vi "Drive.vi"() -> ()   [LabVIEW 2012]
uses:
  Robot Global Data.vi
  <vilib>/Rock Robotics/WPI/Joystick/WPI_JoystickGetSetRefNum.vi
  <vilib>/Rock Robotics/WPI/RobotDrive/WPI_RobotDriveGetSetRefNum.vi
  <vilib>/addons/control/pid/pid.llb/PID (DBL).vi
  <vilib>/addons/control/pid/NI_PID_pid.lvlib
panel:
  in  "PID gains":T1={"proportional gain (Kc)"=1.0, "integral time (Ti, min)"=0.01, "derivative time (Td, min)"=0.0} {"derivative time (Td, min)" format="%.3f"; "integral time (Ti, min)" format="%.3f"; "proportional gain (Kc)" format="%.3f"}
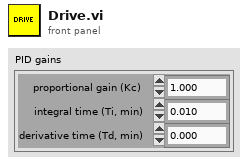
[diagram p1: front panel]
types:
  T1 = cluster{"proportional gain (Kc)":dbl, "integral time (Ti, min)":dbl, "derivative time (Td, min)":dbl}
  T2 = cluster{"Center Position":cluster{"X":dbl, "Y":dbl}, "Distance (ft)":dbl, "Center":bool}[]
  T3 = cluster{"Target Info[0]":cluster{"Center Position":cluster{"X":dbl, "Y":dbl}, "Distance (ft)":dbl, "Center":bool}, "Target Info[1]":cluster{"Center Position":cluster{"X":dbl, "Y":dbl}, "Distance (ft)":dbl, "Center":bool}, "Target Info[2]":cluster{"Center Position":cluster{"X":dbl, "Y":dbl}, "Distance (ft)":dbl, "Center":bool}, "Target Info[3]":cluster{"Center Position":cluster{"X":dbl, "Y":dbl}, "Distance (ft)":dbl, "Center":bool}, "Target Info[4]":cluster{"Center Position":cluster{"X":dbl, "Y":dbl}, "Distance (ft)":dbl, "Center":bool}, "Target Info[5]":cluster{"Center Position":cluster{"X":dbl, "Y":dbl}, "Distance (ft)":dbl, "Center":bool}, "Target Info[6]":cluster{"Center Position":cluster{"X":dbl, "Y":dbl}, "Distance (ft)":dbl, "Center":bool}, "Target Info[7]":cluster{"Center Position":cluster{"X":dbl, "Y":dbl}, "Distance (ft)":dbl, "Center":bool}, "Target Info[8]":cluster{"Center Position":cluster{"X":dbl, "Y":dbl}, "Distance (ft)":dbl, "Center":bool}}
  T4 = cluster{"Center Position":cluster{"X":dbl, "Y":dbl}, "Distance (ft)":dbl, "Center":bool}
  T5 = typedef "WPI_JoystickDevRef.ctl" = cluster{"Device":T6}
  T6 = typedef "WPI_JoystickDeviceEnum.ctl" = enum16{"USB 1", "USB 2", "USB 3", "USB 4", "Kinect 1", "Kinect 2"}
  T7 = typedef "WPI_JoystickButtonState.ctl" = cluster{"Button 1":bool, "Button 2":bool, "Button 3":bool, "Button 4":bool, "Button 5":bool, "Button 6":bool, "Button 7":bool, "Button 8":bool, "Button 9":bool, "Button 10":bool, "Button 11":bool, "Button 12":bool}
  T8 = cluster{"axis 1 (x)":dbl, "axis 2 (y)":dbl, "axis 3 (throttle)":dbl, "axis 4":dbl, "axis 5":dbl, "axis 6":dbl}
  T9 = typedef "WPI_RobotDriveDevRef.ctl" = cluster{"DevStatus":errorcluster, "Motors[]":T10[], "Square Inputs":bool, "Max Output":dbl, "Isochronous":bool}
  T10 = typedef "WPI_MotorControlDeviceRef.ctl" = cluster{"DeviceStatus":errorcluster, "Type":enum16{"PWM", "CAN"}, "PWM":cluster{"Digital Module":T11, "PWM Channel":T12, "DeadBand":T13}, "CAN":cluster{"Device Number":u8, "Control Mode":T14, "Semaphore":T15, "Max Vout":dbl}, "Invert":bool, "TransformRef":T16, "InvTransformRef":T16}
  T11 = typedef "FPGA_TypedefDigitalModule.ctl" = enum16{"Digital Module 1", "Digital Module 2"}
  T12 = typedef "FPGA_DIOPWMChannel.ctl" = enum8{"PWM 1", "PWM 2", "PWM 3", "PWM 4", "PWM 5", "PWM 6", "PWM 7", "PWM 8", "PWM 9", "PWM 10", "Invalid"}
  T13 = typedef "WPI_PWMDeadband.ctl" = cluster{"Name":string, "maxPositivePwm":i32, "minPositivePwm":i32, "centerPwm":i32, "maxNegativePwm":i32, "minNegativePwm":i32, "angularRange":u16}
  T14 = typedef "WPI_CANJaguar_ControlMode.ctl" = enum8{"Percent VBus", "Current", "Speed", "Position", "Voltage"}
  T15 = typedef "Semaphore RefNum" = refnum<k1>
  T16 = typedef "WPI_PWMTransform_ConPane.ctl" = refnum<vi>
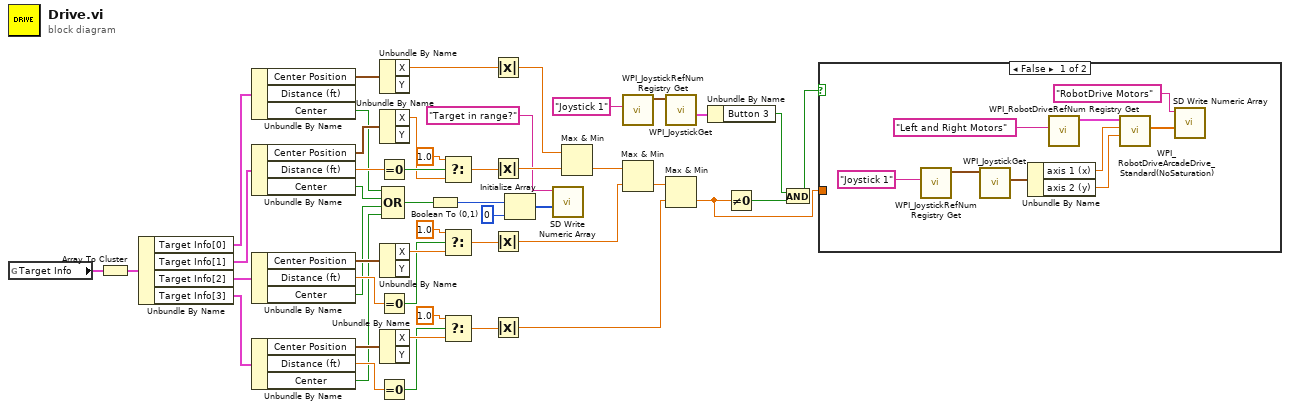
[diagram p0: block diagram]
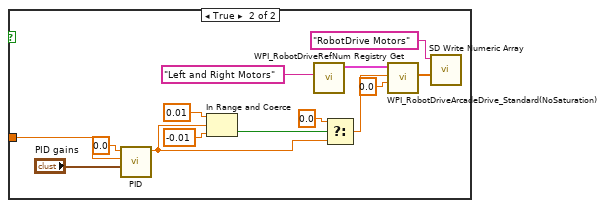
[diagram p2: hidden frame]
diagram:
  n1 = global read "Robot Global Data.vi" "Target Info"() -> (w48:T2)
  n2 = Array To Cluster(array=w48) -> (cluster=w47:T3)
  n3 = Unbundle By Name(w47) -> ("Target Info[0]"=w46:T4, "Target Info[1]"=w37:T4, "Target Info[2]"=w36:T4, "Target Info[3]"=w35:T4)
  n4 = Unbundle By Name(w46) -> ("Center Position"=w45:cluster{"X":dbl, "Y":dbl}, "Center"=w9:bool)  [unwired: 1 out]
  n5 = Unbundle By Name(w37) -> ("Center Position"=w40:cluster{"X":dbl, "Y":dbl}, "Distance (ft)"=w29:dbl, "Center"=w8:bool)
  n6 = Unbundle By Name(w36) -> ("Center Position"=w39:cluster{"X":dbl, "Y":dbl}, "Distance (ft)"=w28:dbl, "Center"=w7:bool)
  n7 = Unbundle By Name(w35) -> ("Center Position"=w38:cluster{"X":dbl, "Y":dbl}, "Distance (ft)"=w27:dbl, "Center"=w6:bool)
  n8 = Equal To 0?(x=w29) -> (x = 0?=w23:bool)
  n9 = Equal To 0?(x=w28) -> (x = 0?=w22:bool)
  n10 = Equal To 0?(x=w27) -> (x = 0?=w21:bool)
  n11 = Unbundle By Name(w45) -> ("X"=w26:dbl)  [unwired: 1 out]
  n12 = Unbundle By Name(w40) -> ("X"=w17:dbl)  [unwired: 1 out]
  n13 = Unbundle By Name(w39) -> ("X"=w24:dbl)  [unwired: 1 out]
  n14 = Unbundle By Name(w38) -> ("X"=w25:dbl)  [unwired: 1 out]
  n15 = Compound Arithmetic op=OR(w9, w8, w7, w6) -> (w4:bool)
  n16 = Boolean To (0,1)(Boolean=w4) -> (0, 1=w1:i16)
  n17 = Select(t=1.0, s=w23, f=w17) -> (s? t:f=w16:dbl)
  n18 = Select(t=1.0, s=w22, f=w24) -> (s? t:f=w15:dbl)
  n19 = Select(t=1.0, s=w21, f=w25) -> (s? t:f=w14:dbl)
  n20 = Absolute Value(x=w26) -> (abs(x)=w13:dbl)
  n21 = Absolute Value(x=w16) -> (abs(x)=w12:dbl)
  n22 = Absolute Value(x=w15) -> (abs(x)=w11:dbl)
  n23 = Absolute Value(x=w14) -> (abs(x)=w10:dbl)
  n24 = Initialize Array(w1, 0 ("dimension size")) -> (w2:i16[])
  n25 = call <vilib>:"SD Write Numeric Array.vi"("Numeric Array"=w2, "Name"="Target in range?") -> ()  [unwired: 8 in, 2 out]
  n26 = Max & Min(x=w13, y=w12) -> (min(x,y)=w34:dbl)  [unwired: 1 out]
  n27 = call <vilib>:"WPI_JoystickRefNum Registry Get.vi"("refnum name"="Joystick 1") -> ("JoystickDevRef"=w43:T5)  [unwired: 9 in, 1 out]
  n28 = Max & Min(x=w34, y=w11) -> (min(x,y)=w32:dbl)  [unwired: 1 out]
  n29 = call <vilib>:"WPI_JoystickGet.vi"("JoystickDevRef"=w43) -> ("Buttons"=w42:T7)  [unwired: 4 in, 2 out]
  n30 = Max & Min(x=w32, y=w10) -> (min(x,y)=w33:dbl)  [unwired: 1 out]
  n31 = Unbundle By Name(w42) -> ("Button 3"=w31:bool)
  n32 = Not Equal To 0?(x=w33) -> (x != 0?=w30:bool)
  n33 = And(x=w31, y=w30) -> (x .and. y?=w41:bool)
  n34 = case shown="False" w41 {
    tunnel: w33 -> [_ w64]
    frame False {
      n35 = call <vilib>:"WPI_JoystickRefNum Registry Get.vi"("refnum name"="Joystick 1") -> ("JoystickDevRef"=w52:T5)  [unwired: 1 in, 9 out]
      n36 = call <vilib>:"WPI_JoystickGet.vi"("JoystickDevRef"=w52) -> ("Axes"=w51:T8)  [unwired: 1 in, 5 out]
      n37 = Unbundle By Name(w51) -> ("axis 1 (x)"=w55:dbl, "axis 2 (y)"=w54:dbl)
      n38 = call <vilib>:"WPI_RobotDriveRefNum Registry Get.vi"("refnum name"="Left and Right Motors") -> ("RobotDriveDevRef"=w56:T9)  [unwired: 1 in, 9 out]
      n39 = call <vilib>:"WPI_RobotDriveArcadeDrive_Standard(NoSaturation).vi"("Y axis value"=w54, "X axis value"=w55, "RobotDriveDevRef"=w56) -> ("Motor Values"=w49:dbl[])  [unwired: 1 in, 7 out]
      n40 = call <vilib>:"SD Write Numeric Array.vi"("Numeric Array"=w49, "Name"="RobotDrive Motors") -> ()  [unwired: 8 in, 2 out]
    }
    frame True {
      n41 = call-poly <vilib>:"PID.vi"("PID gains"="PID gains", "process variable"=w64, "setpoint"=0.0 ("process variable")) -> ("output"=w59:dbl)  [unwired: 7 in, 1 out]
      n42 = In Range and Coerce(upper limit=0.01, x=w59, lower limit=-0.01) -> (In Range?=w61:bool)  [unwired: 1 out]
      n43 = call <vilib>:"WPI_RobotDriveRefNum Registry Get.vi"("refnum name"="Left and Right Motors") -> ("RobotDriveDevRef"=w68:T9)  [unwired: 1 in, 9 out]
      n44 = Select(t=0.0, s=w61, f=w59) -> (s? t:f=w58:dbl)
      n45 = call <vilib>:"WPI_RobotDriveArcadeDrive_Standard(NoSaturation).vi"("Y axis value"=0.0, "X axis value"=w58, "RobotDriveDevRef"=w68) -> ("Motor Values"=w67:dbl[])  [unwired: 1 in, 7 out]
      n46 = call <vilib>:"SD Write Numeric Array.vi"("Numeric Array"=w67, "Name"="RobotDrive Motors") -> ()  [unwired: 8 in, 2 out]
    }
  }
